vi "Update Parameters.vi"(8 "error in (no error)":errorcluster, 10 "Parameters":string[][](array[string]), 11 "Run Instance in":refnum<class "Run Instance.lvclass">) -> (0 "error out":errorcluster, 2 "Same Values":bool, 3 "Run Instance out":refnum<class "Run Instance.lvclass">)   [LabVIEW 2020, in "TALOS.lvlib" / "Run Utilities.lvlib" / "Run Instance.lvclass"]
doc: "Append new parameters or update existing parameters. This VI won't delete parameters from the Run Instance. Providing a list of parameters without a specific parameter will result with the value for the parameter being unchanged."
uses:
  Run Instance.lvclass
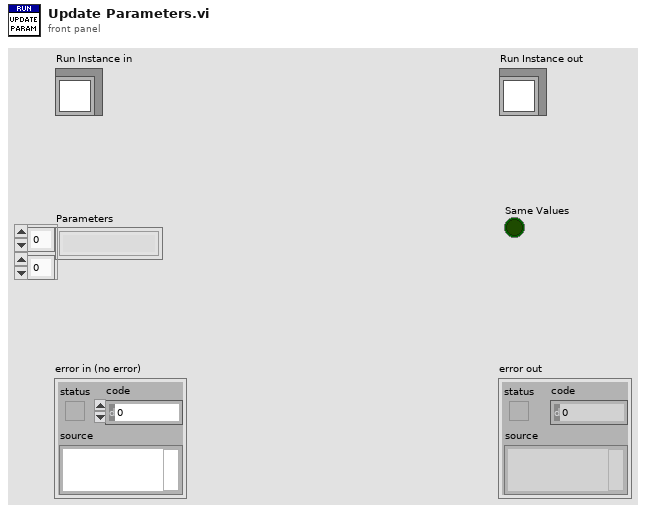
[diagram p1: front panel]
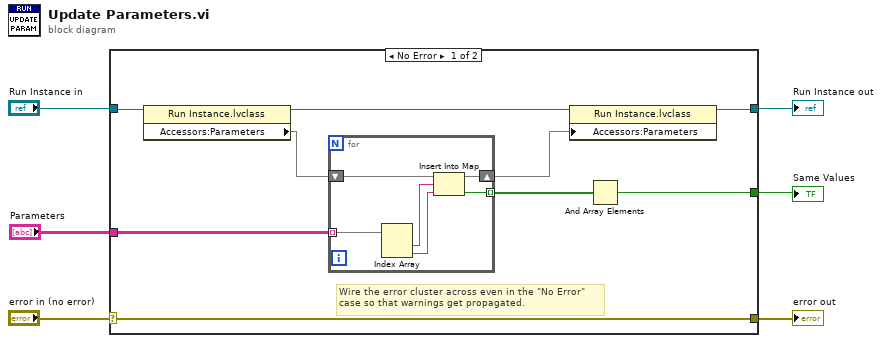
[diagram p0: block diagram]
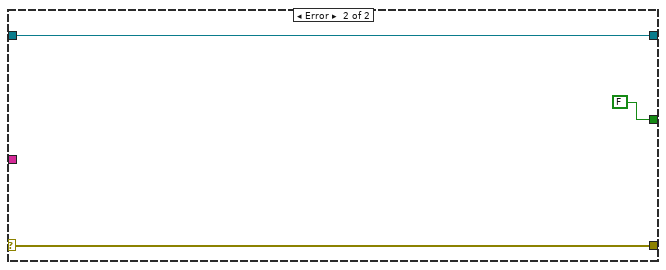
[diagram p2: hidden frame]
diagram:
  n1 = case shown="No Error" "error in (no error)" {
    selector: "error in (no error)" -> [w15 w24]
    tunnel: [w15 w24] -> w5
    tunnel: [w10 w23] -> w3
    tunnel: "Run Instance in" -> [w9 w23]
    tunnel: "Parameters" -> [w8 _]
    tunnel: [w7 FALSE] -> w1
    frame No Error {
      # "Wire the error cluster across even in the \"No Error\"\ncase so that warnings get propagated."
      n2 = property class="Run Instance.lvclass"(reference=w9) -> (reference out=w14:refnum<class "Run Instance.lvclass">, "Accessors:Parameters"=w13:map{string, string})  [unwired: 1 in, 1 out]
      n3 = for {
        tunnel: w8 -> [w19] mode=indexing
        shift-right: [w20] -> w12
        shift-left: w13 -> [w21]
        tunnel: [w16] -> w11 mode=indexing
        n4 = Index Array(array=w19) -> (element #1=w18:string, element #2=w17:string)  [unwired: 2 in]
        n5 = Insert Into Map(map in=w21, key=w18, value=w17) -> (map out=w20:map{string, string}, value unchanged?=w16:bool)  [unwired: 1 out]
      }
      n6 = property class="Run Instance.lvclass"(reference=w14, "Accessors:Parameters"=w12) -> (reference out=w10:refnum<class "Run Instance.lvclass">)  [unwired: 1 in, 1 out]
      n7 = And Array Elements(Boolean array=w11) -> (logical AND=w7:bool)
    }
    frame Error {
    }
  }
  "error out" <- w5
  "Run Instance out" <- w3
  "Same Values" <- w1
